vi "picoquant_log_data.vi"(8 "error in (no error)":errorcluster, 10 "data_in":T1, 11 "hydraharp in":refnum<class "hydraharp.lvclass">) -> (0 "error out":errorcluster, 2 "data_out":T1, 3 "hydraharp out":refnum<class "hydraharp.lvclass">)   [LabVIEW 2015, in "hydraharp.lvclass"]
uses:
  hydraharp.lvclass
  Picoquant_generic/picoquant_data_tdef.ctl
  hydraharp.lvclass/hydraharp.ctl
  Data Logger Class/data_logger.lvclass
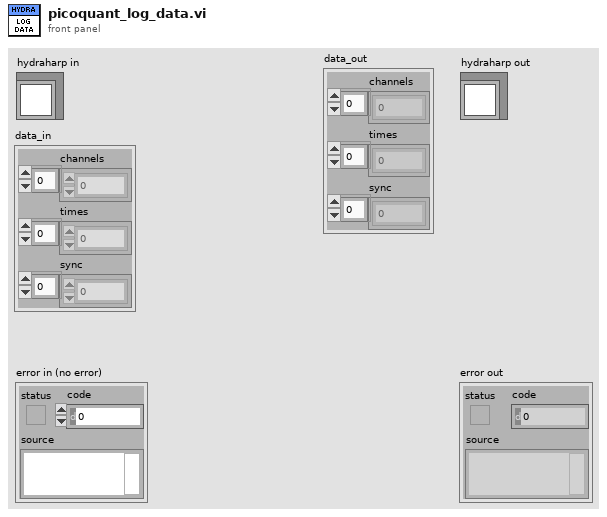
[diagram p1: front panel]
types:
  T1 = typedef "picoquant_data_tdef.ctl" = cluster{"channels":u8[], "times":u64[], "sync":u64[]}
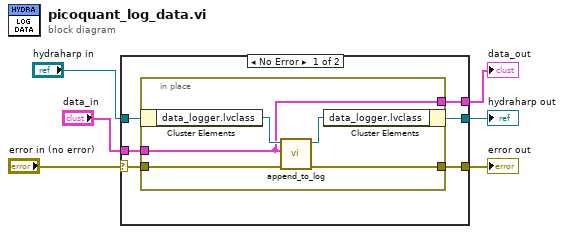
[diagram p0: block diagram]
diagram:
  n1 = case shown="No Error" "error in (no error)" {
    selector: "error in (no error)" -> [w10 w18]
    tunnel: "hydraharp in" -> [w12 w20]
    tunnel: "data_in" -> [w11 w19]
    tunnel: [w9 w18] -> w3
    tunnel: [w8 w19] -> w2
    tunnel: [w7 w20] -> w1
    frame No Error {
      n2 = in-place {
        in-place-border: w11 -> [w13]
        in-place-border: w10 -> [w15]
        in-place-border: [w14] -> w9
        in-place-border: [w13] -> w8
        n3 = in-place-cluster #1(w12) -> ("data_logger.lvclass"=w17:refnum<class "data_logger.lvclass">)
        n4 = call-dynamic "append_to_log.vi"("error in (no error)"=w15, "Data"=w13, "data_logger in"=w17) -> ("error out"=w14:errorcluster, "data_logger out"=w16:refnum<class "data_logger.lvclass">)  [unwired: 7 in]
        n5 = in-place-cluster #1("data_logger.lvclass"=w16) -> (w7:refnum<class "hydraharp.lvclass">)
      }
    }
    frame Error {
    }
  }
  "error out" <- w3
  "hydraharp out" <- w1
  "data_out" <- w2
